vi "LEP_RV_LaunchLoadConfig.vi"(11 "error in (no error)":errorcluster) -> (3 "Connect to a network compile server":bool, 4 "Compiler server name":string, 6 "User name":string, 8 "Password":string, 10 "Remember password":bool, 13 "Secure connection":bool, 14 "Client installed":bool, 15 "error out":errorcluster)   [LabVIEW 2011]
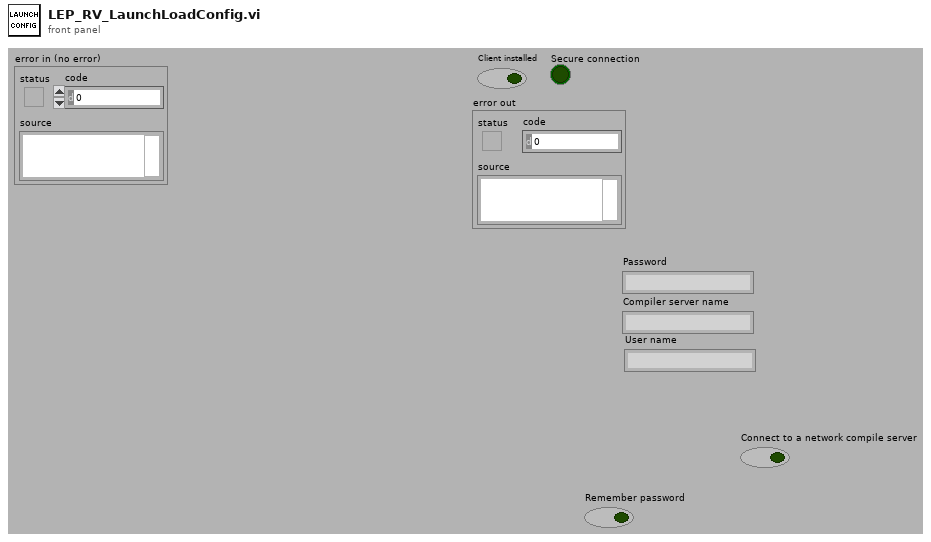
[diagram p1: front panel]
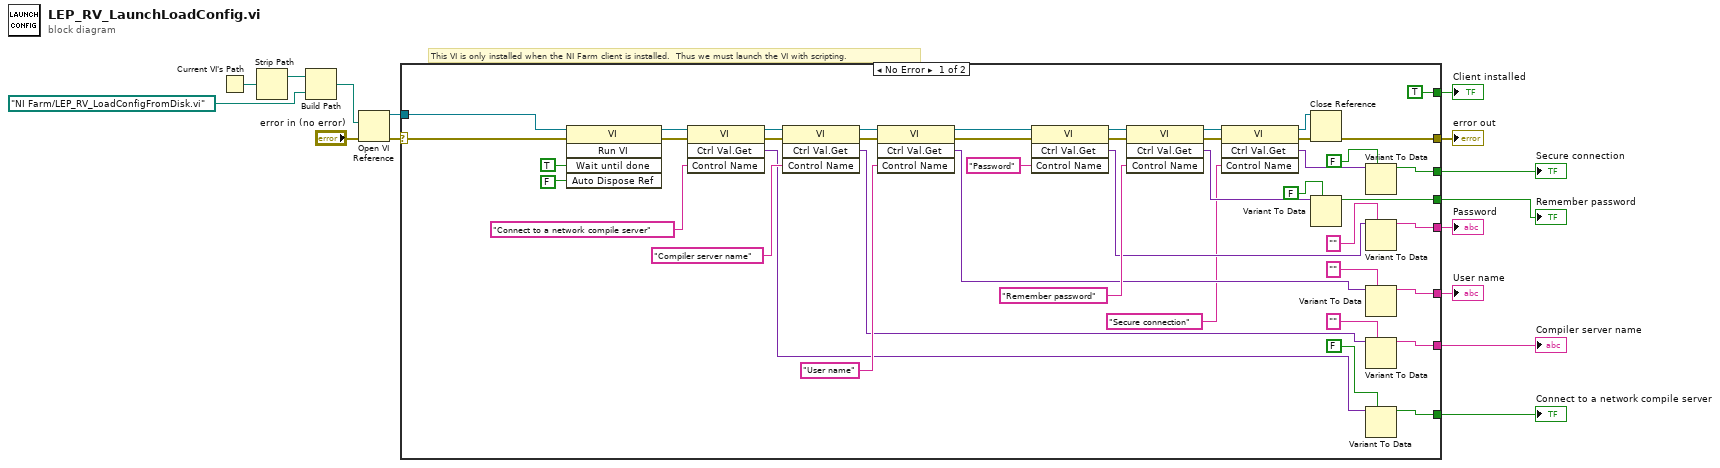
[diagram p0: block diagram]
diagram:
  # "This VI is only installed when the NI Farm client is installed.  Thus we must launch the VI with scripting."
  n1 = Current VI's Path() -> (path=w14:path)
  n2 = Strip Path(path=w14) -> (stripped path=w13:path)  [unwired: 1 out]
  n3 = Build Path(base path=w13, name or relative path=path "NI Farm/LEP_RV_LoadConfigFromDisk.vi") -> (appended path=w12:path)
  n4 = Open VI Reference(vi path=w12, error in (no error)="error in (no error)") -> (vi reference=w11:refnum<vi>, error out=w10:errorcluster)  [unwired: 4 in]
  n5 = case shown="No Error" w10 {
    selector: w10 -> [w54 _]
    tunnel: w11 -> [w59 _]
    tunnel: [w30 _] -> w9
    tunnel: [w29 _] -> w8
    tunnel: [w28 _] -> w7
    tunnel: [w27 _] -> w6
    tunnel: [w26 _] -> w5
    tunnel: [TRUE _] -> w4
    tunnel: [w24 _] -> w2
    tunnel: [w16 _] -> w1
    frame No Error {
      n6 = invoke class="VI" method="Run VI"(reference=w59, error in=w54, "Wait until done"=TRUE ("Wait Until Done"), "Auto Dispose Ref"=FALSE ("Auto Dispose Reference")) -> (reference out=w56:refnum<vi>, error out=w55:errorcluster)  [unwired: 1 in, 3 out]
      n7 = invoke class="VI" method="Ctrl Val.Get"(reference=w56, error in=w55, "Control Name"="Connect to a network compile server") -> (reference out=w47:refnum<vi>, error out=w46:errorcluster, "Get Control Value Variant"=w35:variant)  [unwired: 1 in, 1 out]
      n8 = invoke class="VI" method="Ctrl Val.Get"(reference=w47, error in=w46, "Control Name"="Compiler server name") -> (reference out=w49:refnum<vi>, error out=w48:errorcluster, "Get Control Value Variant"=w34:variant)  [unwired: 1 in, 1 out]
      n9 = invoke class="VI" method="Ctrl Val.Get"(reference=w49, error in=w48, "Control Name"="User name") -> (reference out=w53:refnum<vi>, error out=w52:errorcluster, "Get Control Value Variant"=w33:variant)  [unwired: 1 in, 1 out]
      n10 = invoke class="VI" method="Ctrl Val.Get"(reference=w53, error in=w52, "Control Name"="Password") -> (reference out=w51:refnum<vi>, error out=w50:errorcluster, "Get Control Value Variant"=w32:variant)  [unwired: 1 in, 1 out]
      n11 = invoke class="VI" method="Ctrl Val.Get"(reference=w51, error in=w50, "Control Name"="Remember password") -> (reference out=w23:refnum<vi>, error out=w21:errorcluster, "Get Control Value Variant"=w31:variant)  [unwired: 1 in, 1 out]
      n12 = invoke class="VI" method="Ctrl Val.Get"(reference=w23, error in=w21, "Control Name"="Secure connection") -> (reference out=w22:refnum<vi>, error out=w20:errorcluster, "Get Control Value Variant"=w18:variant)  [unwired: 1 in, 1 out]
      n13 = Close Reference(reference=w22, error in (no error)=w20) -> (error out=w24:errorcluster)
      n14 = Variant To Data(type=FALSE ("Remember password"), Variant=w31) -> (data=w26:bool)  [unwired: 1 in, 1 out]
      n15 = Variant To Data(type=FALSE ("Secure connection"), Variant=w18) -> (data=w16:bool)  [unwired: 1 in, 1 out]
      n16 = Variant To Data(type="" ("Password"), Variant=w32) -> (data=w27:string)  [unwired: 1 in, 1 out]
      n17 = Variant To Data(type="" ("User name"), Variant=w33) -> (data=w28:string)  [unwired: 1 in, 1 out]
      n18 = Variant To Data(type="" ("Compiler server name"), Variant=w34) -> (data=w29:string)  [unwired: 1 in, 1 out]
      n19 = Variant To Data(type=FALSE ("Connect to a network compile server"), Variant=w35) -> (data=w30:bool)  [unwired: 1 in, 1 out]
    }
    frame Error {
    }
  }
  "Password" <- w6
  "Compiler server name" <- w8
  "Connect to a network compile server" <- w9
  "Remember password" <- w5
  "User name" <- w7
  "Client installed" <- w4
  "error out" <- w2
  "Secure connection" <- w1
